vi "Tecan Set Valve.vi"(0 "VISA resource name":refnum<visa-resource-name>="COM3", 1 "Pump Address":T2, 5 "Valve":T1, 11 "error IO":errorcluster) -> (4 "VISA resource name out":refnum<visa-resource-name>, 8 "Error Code":string, 10 "Move Successful":bool, 14 "Response":string, 15 "error out":errorcluster)   [LabVIEW 2020]
uses:
  Pump Address.ctl
  Valve selector.ctl
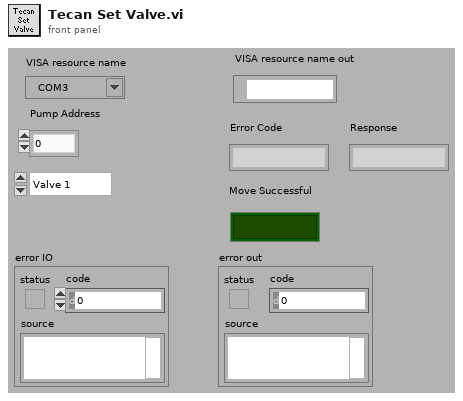
[diagram p1: front panel]
types:
  T1 = typedef "Valve selector.ctl" = enum16{"Valve 1", "Valve 2", "Valve 3", "Valve 4", "Valve 5", "Valve 6", "Valve 7", "Valve 8", "Valve 9"}
  T2 = typedef "Pump Address.ctl" = enum16{"0", "1", "2", "3", "4", "5", "6", "7"}
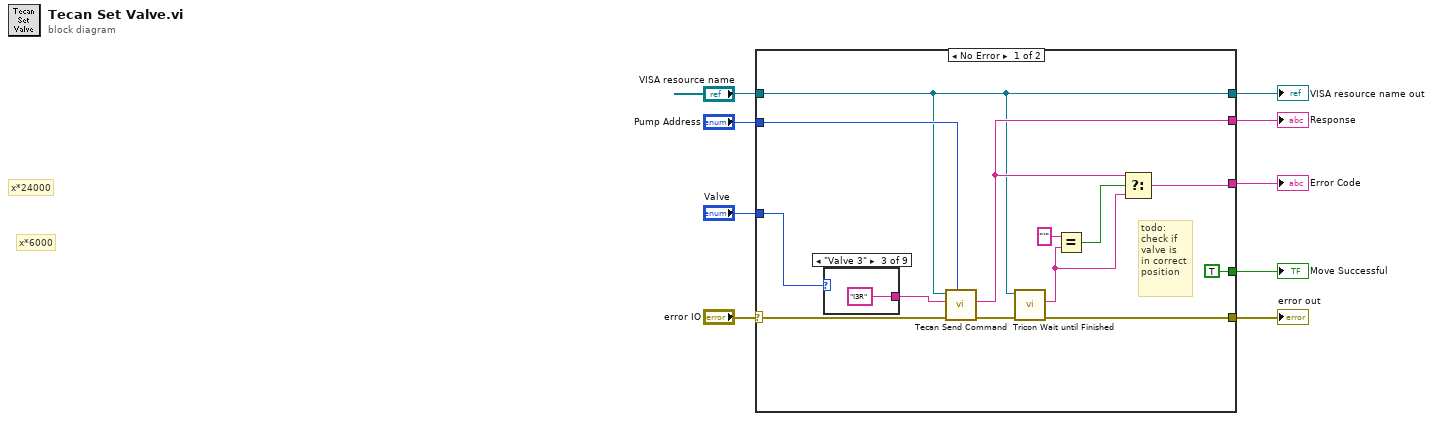
[diagram p0: block diagram]
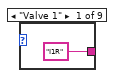
[diagram p2: hidden frame]
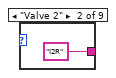
[diagram p3: hidden frame]
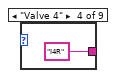
[diagram p4: hidden frame]
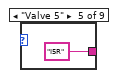
[diagram p5: hidden frame]
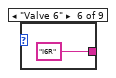
[diagram p6: hidden frame]
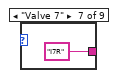
[diagram p7: hidden frame]
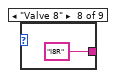
[diagram p8: hidden frame]
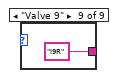
[diagram p9: hidden frame]
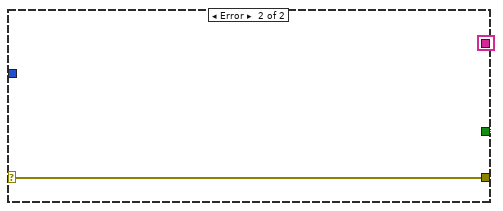
[diagram p10: hidden frame]
diagram:
  # "x*24000"
  # "x*6000"
  n1 = case shown="No Error" "error IO" {
    selector: "error IO" -> [w21 w34]
    tunnel: [w16 w34] -> w9
    tunnel: "Pump Address" -> [w19 _]
    tunnel: "VISA resource name" -> [w10 _]
    tunnel: [TRUE FALSE] -> w6
    tunnel: [w12 ""] -> w5
    tunnel: [w10 _] -> w4
    tunnel: [w14 _] -> w3
    tunnel: "Valve" -> [w18 _]
    frame No Error {
      # "todo:\ncheck if\nvalve is \nin correct\nposition"
      n2 = case shown="\"Valve 3\"" w18 {
        tunnel: ["I1R" ("Command") "I2R" ("Command") "I3R" ("Command") "I4R" ("Command") "I5R" ("Command") "I6R" ("Command") "I7R" ("Command") "I8R" ("Command") "I9R" ("Command")] -> w17
        frame "Valve 1" {
        }
        frame "Valve 2" {
        }
        frame "Valve 3" {
        }
        frame "Valve 4" {
        }
        frame "Valve 5" {
        }
        frame "Valve 6" {
        }
        frame "Valve 7" {
        }
        frame "Valve 8" {
        }
        frame "Valve 9" {
        }
      }
      n3 = call "Tecan Send Command.vi"("Address"=w19, "error in (no error)"=w21, "Command"=w17, "VISA resource name in"=w10) -> ("error out"=w20:errorcluster, "Raw Response"=w14:string)  [unwired: 3 in, 3 out]
      n4 = call "Tricon Wait until Finished.vi"("error out"=w20, "VISA resource name in"=w10) -> ("error out"=w16:errorcluster, "Error Code"=w13:string)  [unwired: 6 in, 2 out]
      n5 = Equal?(x="'", y=w13) -> (x = y?=w15:bool)
      n6 = Select(t=w14, s=w15, f=w13) -> (s? t:f=w12:string)
    }
    frame Error {
    }
  }
  "error out" <- w9
  "VISA resource name out" <- w4
  "Move Successful" <- w6
  "Error Code" <- w5
  "Response" <- w3
